vi "Show Cursors.vi"(6 "Cursor Options":T1={"font"={"Font Name"="Arial", "Size"=14, "Strikeout?"=FALSE, "Italic?"=FALSE, "Underline?"=FALSE, "Outline?"=FALSE, "Shadow?"=FALSE, "Bold?"=FALSE}, "size"=1, "Timestamp"=enum."at TOP", "Vertical Line?"=TRUE, "Horizontal Line?"=TRUE, "alignment(left, top)"={"horizontal"=enum."left", "vertical"=enum."center"}, "TextFormat"=" %3$s\\n %2$.2f", "time format (%H:%M:%S)"="%H:%M:%S"} {"size" min=1 max=50}, 8 "error in (no error)":errorcluster, 9 "Coords":T2, 10 "XY Graph":refnum<vi>, 11 "input picture":picture) -> (0 "error out":errorcluster, 1 "출력 클러스터":cluster{"X":dbl, "Y":dbl}, 3 "output picture":picture)   [LabVIEW 2018]
doc: "Shows real time cursors overlayed in a graph, using just one mouse move event case. The options for the cursors can be highly customized to set up a unique cursor style.\n\nUsage: Place this inside an event structure on any XY graph, in the \"Mouse Move\" event case. Set the options as an input cluster to override the defaults. The output picture control would typically be connected to the XY Graph's \"PlotImages.Front\" property item.\n\nCursor Options\n<b>Horizontal Line?</b> - Draws a horizontal line to intersect each plot\n<b>Verticle Line?</b> - Draws a verticle line at the mouse location to highlight the cursor location (typically on the time scale)\n<b>Timestamp</b> - Sets where to display the timestamp (if you want it at the top or bottom) Used best with the verticle line turned on.\n<b>Font</b> - Setup the font for displaying the cursor text\n<b>Alignment</b> - Sets the alignment options for the text relative to the cursor point\n<b>TextFormat</b> - Sets the text display format at the cursor points to show. Three input parameters are available for the text, which can be accessed using parameter numbers.\ninputs: \n1$ - Timestamp at cursor locations\n2$ - Value of the plot\n3$ - Name of the plot\n\nExamples: $2$.2f\\n\\n%1$s\nThis shows the value of the plot with 2 decimal places. A blank line, then the name of the plot"
uses:
  <vilib>/Utility/miscctls.llb/LVPoint32TypeDef.ctl
  CursorOptions.ctl
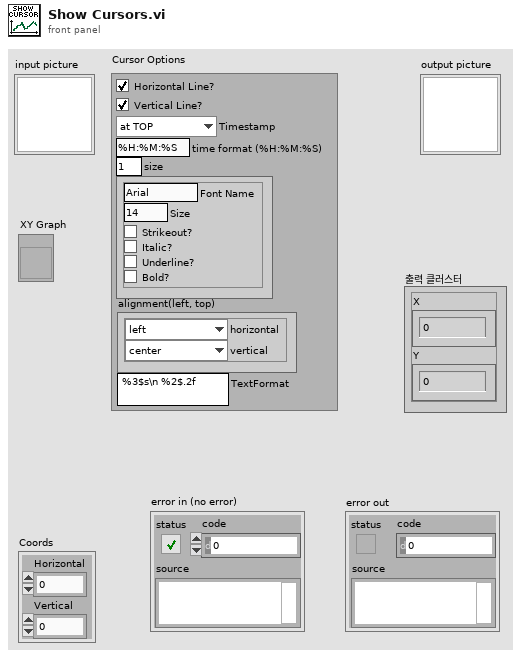
[diagram p1: front panel]
types:
  T1 = typedef "CursorOptions.ctl" = cluster{"font":cluster{"Font Name":string, "Size":i16, "Strikeout?":bool, "Italic?":bool, "Underline?":bool, "Outline?":bool, "Shadow?":bool, "Bold?":bool}, "size":i16, "Timestamp":enum16{"at TOP", "at BOTTOM", "none"}, "Vertical Line?":bool, "Horizontal Line?":bool, "alignment(left, top)":cluster{"horizontal":enum16{"left", "center", "right"}, "vertical":enum16{"top", "center", "bottom"}}, "TextFormat":string, "time format (%H:%M:%S)":string}
  T2 = typedef "LVPoint32TypeDef.ctl" = cluster{"Horizontal":i32, "Vertical":i32}
  T3 = enum16{"User-specified Font", "Application Font", "System Font", "Dialog Font"}
  T4 = cluster{"horizontal":enum16{"left", "center", "right"}, "vertical":enum16{"top", "center", "bottom"}}
  T5 = cluster{"Font Name":string, "Size":i16, "Strikeout?":bool, "Italic?":bool, "Underline?":bool, "Outline?":bool, "Shadow?":bool, "Bold?":bool}
  T6 = typedef "LVRectTypeDef.ctl" = cluster{"Left":i16, "Top":i16, "Right":i16, "Bottom":i16}
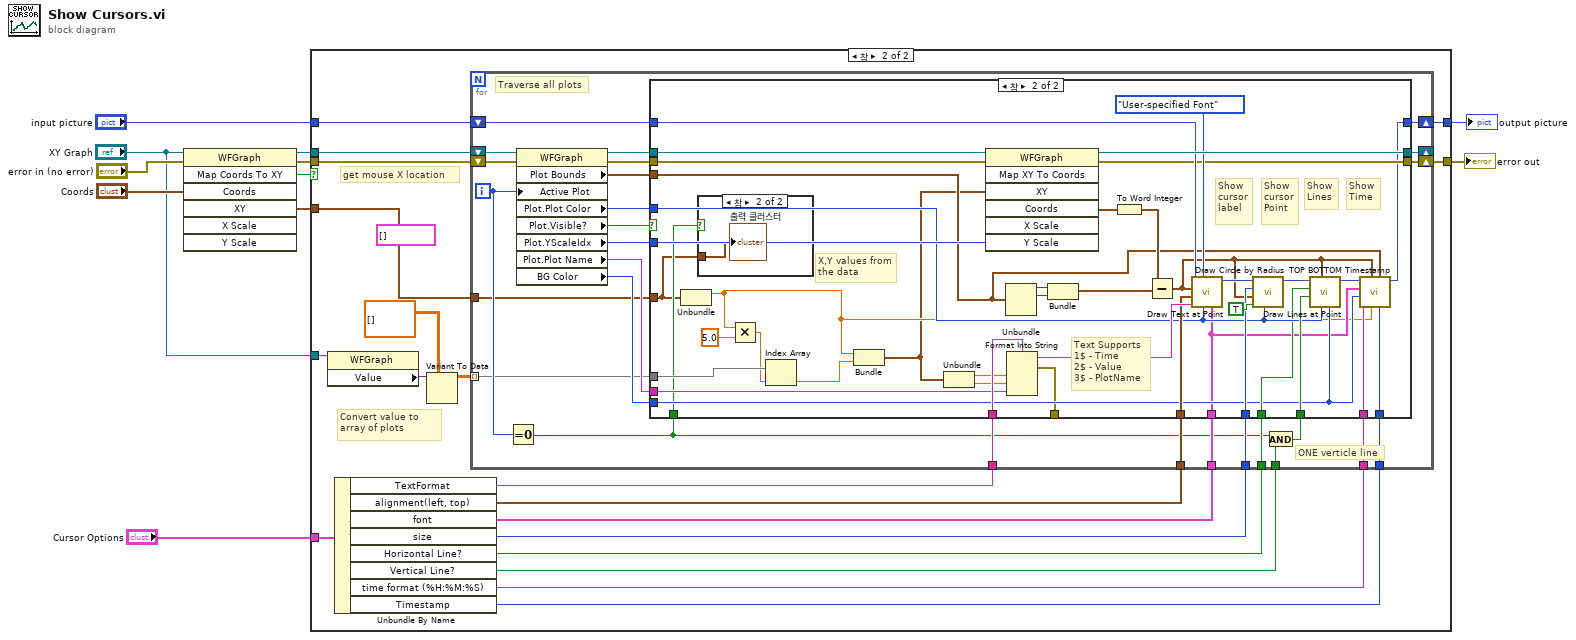
[diagram p0: block diagram]
diagram:
  n1 = invoke on="Invoke Node" class="WFGraph" method="Map Coords To XY"(reference="XY Graph", error in="error in (no error)", "Coords"="Coords") -> (reference out=w8:refnum<vi>, error out=w7:errorcluster, "Map Coords To XY"=w10:bool, "XY"=w11:cluster{"X":dbl, "Y":dbl})  [unwired: 4 in, 3 out]
  n2 = case shown="참" w10 {
    tunnel: w11 -> [_ w31]
    tunnel: w8 -> [_ w32]
    tunnel: [w12 w30] -> w3
    tunnel: w7 -> [w13 w29]
    tunnel: [w13 w28] -> w6
    tunnel: "input picture" -> [w12 w27]
    tunnel: "Cursor Options" -> [_ w19]
    tunnel: "XY Graph" -> [_ w17]
    frame False {
      # "not in plot area.  clear the image"
    }
    frame True {
      (unwired) cluster{dbl[], dbl[]}[] []
      # "Convert value to array of plots"
      # "get mouse X location"
      n3 = property class="WFGraph"(reference=w17) -> ("Value"=w16:variant)  [unwired: 1 in, 2 out]
      n4 = Unbundle By Name(w19) -> ("TextFormat"=w26:string, "alignment(left, top)"=w25:T4, "font"=w24:T5, "size"=w23:i16, "Horizontal Line?"=w22:bool, "Vertical Line?"=w21:bool, "time format (%H:%M:%S)"=w15:string, "Timestamp"=w20:enum16{"at TOP", "at BOTTOM", "none"})
      n5 = Variant To Data(type=dbl[][] [], Variant=w16) -> (data=w18:dbl[][])  [unwired: 1 in, 1 out]
      n6 = for {
        tunnel: w18 -> [w35] mode=indexing
        shift-right: [w58] -> _
        shift-left: w32 -> [w56]
        tunnel: w31 -> [w36]
        shift-right: [w54] -> w30
        shift-left: w27 -> [w57]
        shift-right: [w49] -> w28
        shift-left: w29 -> [w51]
        tunnel: w23 -> [w47]
        tunnel: w25 -> [w46]
        tunnel: w24 -> [w45]
        tunnel: w26 -> [w44]
        tunnel: w22 -> [w43]
        tunnel: w21 -> [w40]
        tunnel: w20 -> [w38]
        tunnel: w15 -> [w34]
        i -> [w42]
        # "Traverse all plots"
        # "ONE verticle line"
        n7 = Equal To 0?(x=w42) -> (x = 0?=w33:bool)
        n8 = property on="Property Node" class="WFGraph"(reference=w56, error in=w51, "Active Plot"=w42) -> (reference out=w55:refnum<vi>, error out=w50:errorcluster, "Plot Bounds"=w59:T6, "Plot.Plot Color"=w53:u32, "Plot.Visible?"=w52:bool, "Plot.YScaleIdx"=w48:u32, "Plot.Plot Name"=w39:string, "BG Color"=w37:u32)
        n9 = And(x=w33, y=w40) -> (x .and. y?=w41:bool)
        n10 = case shown="참" w52 {
          tunnel: w59 -> [_ w75]
          tunnel: [w62 w99] -> w58
          tunnel: w35 -> [_ w70]
          tunnel: w36 -> [_ w63]
          tunnel: w57 -> [w61 w98]
          tunnel: w55 -> [w62 w96]
          tunnel: [w61 w79] -> w54
          tunnel: w53 -> [_ w84]
          tunnel: w50 -> [w60 w92]
          tunnel: [w60 w91] -> w49
          tunnel: w48 -> [_ w90]
          tunnel: w47 -> [_ w89]
          tunnel: w46 -> [_ w88]
          tunnel: w45 -> [_ w73]
          tunnel: w44 -> [_ w87]
          tunnel: w43 -> [_ w83]
          tunnel: w41 -> [_ w86]
          tunnel: w39 -> [_ w80]
          tunnel: w38 -> [_ w77]
          tunnel: w37 -> [_ w74]
          tunnel: [_ w72] -> _
          tunnel: w34 -> [_ w71]
          tunnel: w33 -> [_ w66]
          frame False {
            # "plot is not visible, so don't show the cursor for it."
          }
          frame True {
            # "Show\nTime"
            # "Show\nLines"
            # "Show\ncursor\nPoint"
            # "Show\ncursor\nlabel"
            # "Text Supports\n1$ - Time\n2$ - Value\n3$ - PlotName"
            # "X,Y values from the data"
            n11 = Unbundle(w63) -> ("X"=w69:dbl)  [unwired: 1 out]
            n12 = case shown="참" w66 {
              tunnel: w63 -> [_ w105]
              frame False {
              }
              frame True {
                "출력 클러스터" <- w105
              }
            }
            n13 = Multiply(x=w69, y=5.0) -> (x*y=w68:dbl)
            n14 = Index Array(array=w70, index=w68) -> (element=w65:dbl)
            n15 = Bundle("X"=w69, w65) -> (w64:cluster{"X":dbl, dbl})  [unwired: 1 in]
            n16 = Unbundle(w64) -> ("X"=w82:dbl, w81:dbl)
            n17 = invoke on="Invoke Node" class="WFGraph" method="Map XY To Coords"(reference=w96, error in=w92, "XY"=w64, "Y Scale"=w90) -> (reference out=w99:refnum<vi>, error out=w91:errorcluster, "Coords"=w104:T2)  [unwired: 3 in, 4 out]
            n18 = Unbundle(w75) -> ("Left"=w102:i16, "Top"=w103:i16)  [unwired: 2 out]
            n19 = Format Into String(format string=w87, w82, w81, w80) -> (resulting string=w97:string, error out=w72:errorcluster)  [unwired: 2 in]
            n20 = Bundle("Left"=w102, "Top"=w103) -> (w100:cluster{"Left":i16, "Top":i16})  [unwired: 1 in]
            n21 = To Word Integer(number=w104) -> (16bit integer=w101:cluster{"Horizontal":i16, "Vertical":i16})
            n22 = Subtract(x=w101, y=w100) -> (x-y=w76:cluster{i16, i16})
            n23 = call <vilib>:"Draw Text at Point.vi"("[user-specified font]"=w73, "text color(black)"=w84, "desired font(Application)"=T3."User-specified Font", "text"=w97, "alignment(left, top)"=w88, "origin"=w76, "picture"=w98) -> ("new picture"=w95:picture)  [unwired: 3 in, 1 out]
            n24 = call <vilib>:"Draw Circle by Radius.vi"("color(black)"=w84, "fill?(F)"=TRUE, "pixel center"=w76, "radius"=w89, "picture"=w95) -> ("new picture"=w85:picture)  [unwired: 6 in]
            n25 = call "Draw Lines at Point.vi"("GraphBGK"=w74, "color(black)"=w84, "pixel center"=w76, "Vertical Line?"=w86, "Horizontal Line?"=w83, "new picture in"=w85) -> ("new picture out"=w78:picture)  [unwired: 5 in]
            n26 = call "TOP BOTTOM Timestamp.vi"("Format"=w77, "Rect"=w75, "Timestamp"=w69, "pixel center"=w76, "time format (%H:%M:%S)"=w71, "GraphBGK"=w74, "font"=w73, "new picture in"=w78) -> ("new picture out"=w79:picture)  [unwired: 3 in]
          }
        }
      }
    }
  }
  "error out" <- w6
  "output picture" <- w3
